vi "teszt_sampling_error.vi"() -> ()   [LabVIEW 2014]
panel:
  out "Phase":cluster{i32[], dbl[]}(graph)
  out "Mag":cluster{i32[], dbl[]}(graph)
  out "actual s":i32
  out "elemszam korlat":dbl
  out "real fs [Hz]":dbl
  out "Waveform Graph":waveform(dbl)[](graph)
  out "Phase":dbl
  out "Mag":dbl
  out "tmr 2 rld value":u16
  in  "Signal freq [Hz]":u32=1000
  out "VISA Refnum out":refnum<visa-resource-name>
  out "error out":errorcluster
  in  "VISA Refnum in":refnum<visa-resource-name>
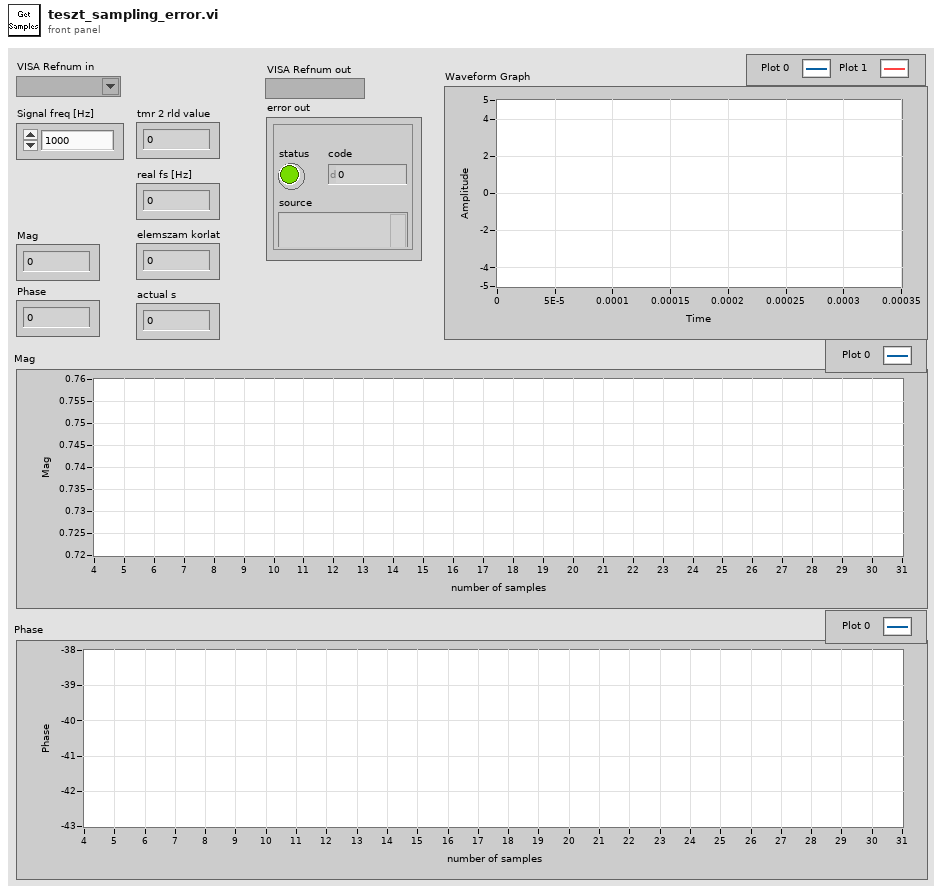
[diagram p1: front panel]
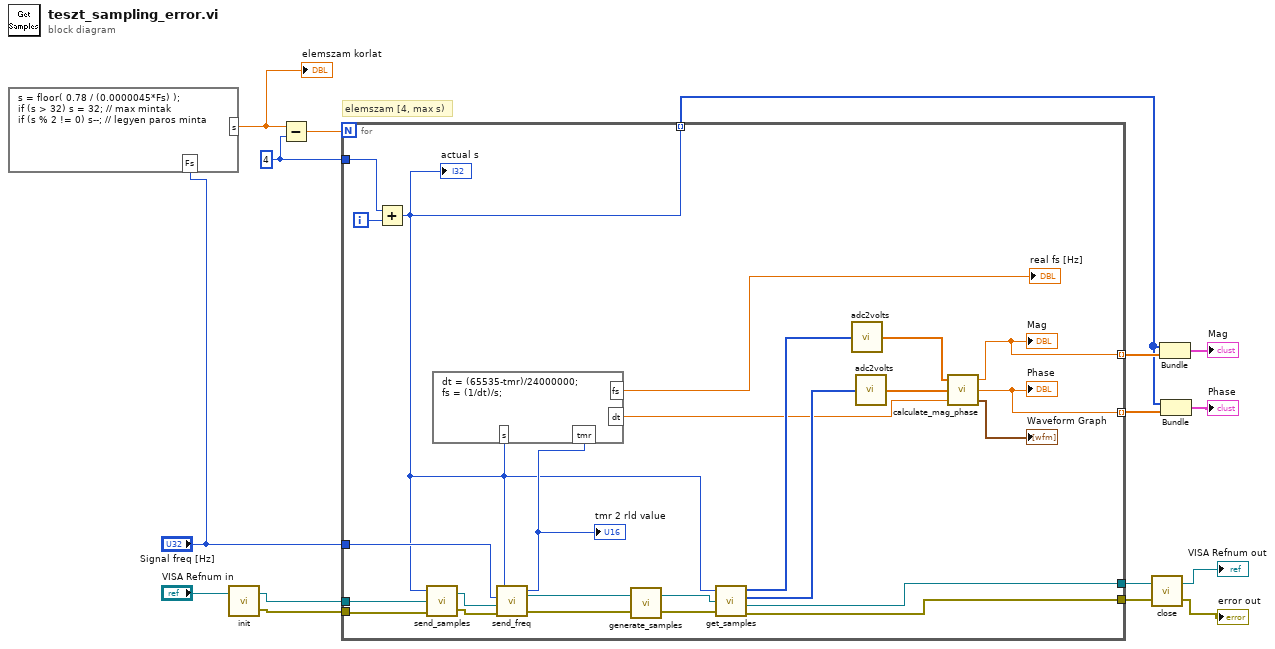
[diagram p0: block diagram]
diagram:
  w1 = 4 ("x")
  # "elemszam [4, max s)"
  n1 = formula code="s = floor( 0.78 / (0.0000045*Fs) );\nif (s > 32) s = 32; // max mintak\nif (s % 2 != 0) s--; // legyen paros minta"("Fs"="Signal freq [Hz]") -> ("s"=w2:dbl)
  "elemszam korlat" <- w2
  n2 = call "init.vi"("VISA Refnum in"="VISA Refnum in") -> ("error out"=w12:errorcluster, "VISA Refnum out"=w13:refnum<visa-resource-name>)  [unwired: 1 in]
  n3 = Subtract(x=w2, y=w1) -> (x-y=w9:dbl)
  n4 = for {
    N: w9 -> [_]
    tunnel: "Signal freq [Hz]" -> [w37]
    tunnel: w13 -> [w27]
    tunnel: w12 -> [w26]
    tunnel: [w25] -> w11
    tunnel: [w24] -> w10
    tunnel: [w21] -> w7 mode=indexing
    tunnel: [w20] -> w5 mode=indexing
    tunnel: [w18] -> w6 mode=indexing
    tunnel: w1 -> [w17]
    i -> [w19]
    n5 = Add(x=w17, y=w19) -> (x+y=w18:i32)
    "actual s" <- w18
    n6 = call "send_samples.vi"("error in (no error)"=w26, "VISA Refnum in"=w27, "elemszam"=w18) -> ("error out"=w34:errorcluster, "VISA Refnum out"=w35:refnum<visa-resource-name>)
    n7 = call "send_freq.vi"("error in (no error)"=w34, "VISA Refnum in"=w35, "signal freq"=w37, "elemszam"=w18) -> ("error out"=w39:errorcluster, "VISA Refnum out"=w38:refnum<visa-resource-name>, "tmr 2 rld value"=w29:u16)
    "tmr 2 rld value" <- w29
    n8 = formula code="dt = (65535-tmr)/24000000;\nfs = (1/dt)/s;"("tmr"=w29, "s"=w18) -> ("dt"=w28:dbl, "fs"=→"real fs [Hz]":dbl)
    n9 = call "generate_samples.vi"("error in (no error)"=w39, "VISA Refnum in"=w38) -> ("error out"=w40:errorcluster, "VISA Refnum out"=w36:refnum<visa-resource-name>)
    n10 = call "get_samples.vi"("elemszam"=w18, "VISA Refnum in"=w36, "error in (no error)"=w40) -> ("in samples"=w33:u16[], "out samples"=w32:u16[], "VISA Refnum out"=w25:refnum<visa-resource-name>, "error out"=w24:errorcluster)
    n11 = call "adc2volts.vi"("ADC value"=w33) -> ("Volts"=w31:dbl[])
    n12 = call "adc2volts.vi"("ADC value"=w32) -> ("Volts"=w30:dbl[])
    n13 = call "calculate_mag_phase.vi"("dt"=w28, "OUT samples"=w30, "IN samples"=w31) -> ("Measured Signals"=→"Waveform Graph":waveform(dbl)[], "Phase"=w20:dbl, "Magnitude"=w21:dbl)
    "Mag" <- w21
    "Phase" <- w20
  }
  n14 = call "close.vi"("error in (no error)"=w10, "VISA resource name"=w11) -> ("error out"=→"error out":errorcluster, "VISA resource name out"=→"VISA Refnum out":refnum<visa-resource-name>)
  n15 = Bundle(w6, w7) -> (→"Mag":cluster{i32[], dbl[]})  [unwired: 1 in]
  n16 = Bundle(w6, w5) -> (→"Phase":cluster{i32[], dbl[]})  [unwired: 1 in]
